vi "Calibration.vi"() -> ()   [LabVIEW 2021]
uses:
  C:/Users/User/Documents/CB III control files/Thorlabs.MotionControl.Controls.dll
  CB III control files/Thorlabs.MotionControl.Controls.dll
  C:/Users/User/Documents/CB III control files/ThorLabs.MotionControl.Benchtop.DCServoCLI.dll
  CB III control files/ThorLabs.MotionControl.Benchtop.DCServoCLI.dll
  C:/Users/User/Documents/CB III control files/ThorLabs.MotionControl.KCube.DCServoCLI.dll
  CB III control files/ThorLabs.MotionControl.KCube.DCServoCLI.dll
  C:/Users/User/Documents/CB III control files/Thorlabs.MotionControl.IntegratedStepperMotorsCLI.dll
  CB III control files/Thorlabs.MotionControl.IntegratedStepperMotorsCLI.dll
  <vilib>/Utility/file.llb/Read Delimited Spreadsheet (DBL).vi
  <vilib>/Utility/file.llb/Write Delimited Spreadsheet (DBL).vi
  <vilib>/ptbypt/NI_PtbyPt.lvlib
panel:
  in  "Drill camera#":dbl=1.0
  in  "OCT camera#":dbl=2.0
  out "sensitivity":dbl
  out "pilot_radii":dbl[][](array[numeric])
  out "pilot_centers":dbl[][](array[numeric])
  out "Targets in OCT":dbl[][](array[numeric])
  in  "take pic":bool
  out "Lumedica report 3":string
  in  "saveing method 3":string(combo)="SaveQueueImages"
  in  "USB camera calibration":bool
  out "OCT ON":bool=TRUE
  out "Lumedica report":string
  in  "saveing method":string(combo)="SaveQueueImages"
  in  "?":bool
  out "OCT imaging position":dbl[](array[numeric])
  in  "?":bool
  out "all pilot points":dbl[][](array[numeric])
  in  "Relative pilot points path":path=path "C:/Users/User/Documents/CB III control files/pilotpoints2.txt"
  in  "?":bool
  out "X-stage Control":refnum<k24>
  out "X stage properties":refnum<k24>
  in  "LongTravelStageControl":refnum<k24>(container)
  out "Zero Position":dbl[](array[numeric])
  out "Drill-Z-stage Control":refnum<k24>
  out "OCT-Z-stage-control":refnum<k24>
  out "Y-stage Control":refnum<k24>
  out "Y-stage properties":refnum<k24>
  out "Driller-Z-stage-Properties":refnum<k24>
  out "OCT-Z stage-properites":refnum<k24>
  in  "Trajectory":dbl[][](array[numeric])
  out "Velocity":T1(graph)
  out "position":T1(graph)
  in  "Driller Z- stage":refnum<k24>(container)
  in  "Y stage":refnum<k24>(container)
  in  "OCT Z-stage":refnum<k24>(container)
  # "USB Camera calibration"
  # "Constant trench depth on skull updates"
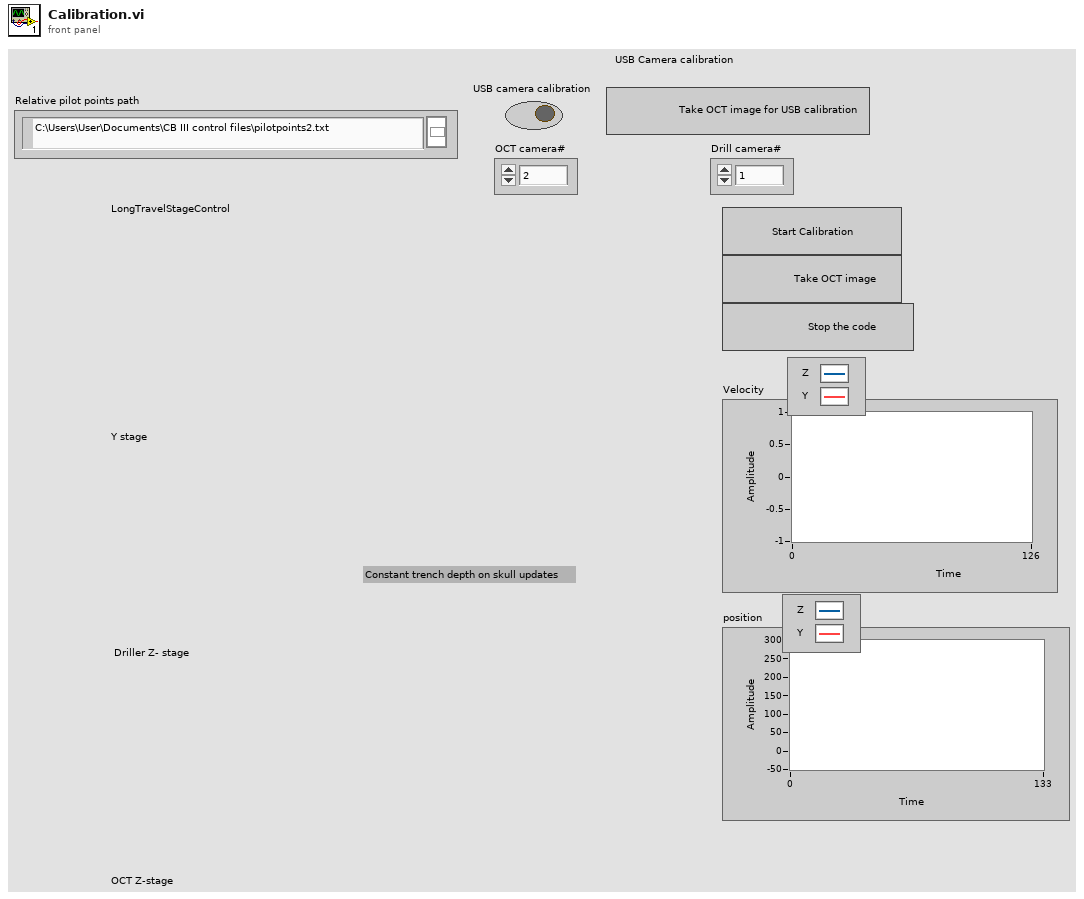
[diagram p1: front panel]
types:
  T1 = cluster{"[0]":dbl, "[1]":dbl, "[2]":dbl, "[3]":dbl, "[4]":dbl, "[5]":dbl, "[6]":dbl, "[7]":dbl, "[8]":dbl}
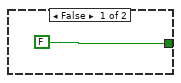
[diagram p3: hidden frame]
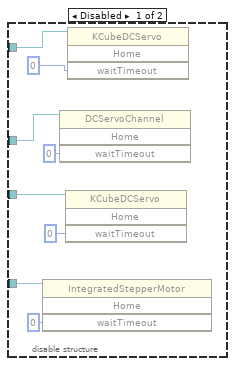
[diagram p4: hidden frame]
diagram:
  n1 = flat-sequence {
    tunnel: [w78] -> w5
    tunnel: w5 -> [w93]
    tunnel: [w211] -> w2
    tunnel: w2 -> [w216]
    tunnel: [w223] -> w4
    tunnel: [w222] -> w3
    tunnel: w4 -> [w225]
    tunnel: w3 -> [w224]
    frame #0 {
      # "Initiate all actuators"
      # "Initiate all actuators"
      n2 = property class="KCubeDCServoControl"(reference="Driller Z- stage", "SerialNumber"="27260819") -> (reference out=w39:refnum<k24>)  [unwired: 1 in, 1 out]
      n3 = property class="LongTravelStageControl"(reference="LongTravelStageControl", "SerialNumber"="45285094") -> (reference out=w28:refnum<k24>)  [unwired: 1 in, 1 out]
      n4 = property class="BenchtopDCServoControl"(reference="Y stage", "SerialNumber"="105278474") -> (reference out=w36:refnum<k24>)  [unwired: 1 in, 1 out]
      n5 = property class="KCubeDCServoControl"(reference="OCT Z-stage", "SerialNumber"="27261776") -> (reference out=w43:refnum<k24>)  [unwired: 1 in, 1 out]
      n6 = invoke class="KCubeDCServoControl" method="CreateDevice"(reference=w39) -> (reference out=w20:refnum<k24>)  [unwired: 2 in, 2 out]
      n7 = invoke class="LongTravelStageControl" method="CreateDevice"(reference=w28) -> (reference out=w27:refnum<k24>)  [unwired: 2 in, 2 out]
      n8 = invoke class="KCubeDCServoControl" method="CreateDevice"(reference=w43) -> (reference out=w18:refnum<k24>)  [unwired: 2 in, 2 out]
      n9 = invoke class="BenchtopDCServoControl" method="CreateDevice"(reference=w36) -> (reference out=w34:refnum<k24>)  [unwired: 2 in, 2 out]
      n10 = property class="KCubeDCServoControl"(reference=w18) -> (reference out=w33:refnum<k24>, "Device"=w16:refnum<k24>)  [unwired: 1 in, 1 out]
      n11 = local write "OCT-Z stage-properites"(w33) -> ()
      n12 = property class="LongTravelStageControl"(reference=w27) -> (reference out=w26:refnum<k24>, "Device"=w25:refnum<k24>)  [unwired: 1 in, 1 out]
      n13 = invoke class="IntegratedStepperMotor" method="SetBacklash"(reference=w25, "backlash"=0.002) -> ()  [unwired: 2 in, 4 out]
      n14 = property class="KCubeDCServoControl"(reference=w20) -> (reference out=w32:refnum<k24>, "Device"=w17:refnum<k24>)  [unwired: 1 in, 1 out]
      n15 = property class="BenchtopDCServoControl"(reference=w34) -> (reference out=w31:refnum<k24>, "BenchtopDCServo"=w23:refnum<k24>)  [unwired: 1 in, 1 out]
      n16 = invoke class="DCServoChannel" method="SetBacklash"(reference=w23, "backlash"=0.0) -> ()  [unwired: 2 in, 4 out]
      n17 = invoke class="IntegratedStepperMotor" method="EnableDevice"(reference=w25) -> ()  [unwired: 2 in, 3 out]
      n18 = invoke class="DCServoChannel" method="EnableDevice"(reference=w23) -> ()  [unwired: 2 in, 3 out]
      n19 = invoke class="KCubeDCServo" method="SetBacklash"(reference=w17, "backlash"=0.007) -> ()  [unwired: 2 in, 4 out]
      n20 = invoke class="KCubeDCServo" method="SetBacklash"(reference=w16, "backlash"=0.007) -> ()  [unwired: 2 in, 4 out]
      n21 = local write "OCT-Z-stage-control"(w16) -> ()
      n22 = local write "Driller-Z-stage-Properties"(w32) -> ()
      n23 = local write "Drill-Z-stage Control"(w17) -> ()
      n24 = local write "X stage properties"(w26) -> ()
      n25 = local write "X-stage Control"(w25) -> ()
      n26 = local write "Y-stage properties"(w31) -> ()
      n27 = local write "Y-stage Control"(w23) -> ()
    }
    frame #1 {
      # "Home actuators"
      n28 = local read "Drill-Z-stage Control"() -> (w47:refnum<k24>)
      n29 = local read "OCT-Z-stage-control"() -> (w45:refnum<k24>)
      n30 = local read "Y-stage Control"() -> (w46:refnum<k24>)
      n31 = local read "X-stage Control"() -> (w44:refnum<k24>)
      n32 = disable-structure shown="Enabled" {
        disable-tunnel: w46 -> [w55 _]
        disable-tunnel: w47 -> [w53 _]
        disable-tunnel: w45 -> [w51 _]
        disable-tunnel: w44 -> [w49 _]
        frame Disabled {
          n33 = invoke class="IntegratedStepperMotor" method="Home"(reference=w49, "waitTimeout"=0) -> ()  [unwired: 2 in, 4 out]
          n34 = invoke class="DCServoChannel" method="Home"(reference=w55, "waitTimeout"=0) -> ()  [unwired: 2 in, 4 out]
          n35 = invoke class="KCubeDCServo" method="Home"(reference=w51, "waitTimeout"=0) -> ()  [unwired: 2 in, 4 out]
          n36 = invoke class="KCubeDCServo" method="Home"(reference=w53, "waitTimeout"=0) -> ()  [unwired: 2 in, 4 out]
        }
        frame Enabled {
        }
      }
    }
    frame #2 {
      n37 = case shown="True" "USB camera calibration" {
        frame False {
        }
        frame True {
          n38 = flat-sequence {
            frame #0 {
              n39 = local write "OCT ON"(TRUE ("OCT ON")) -> ()
              n40 = Wait (ms)(milliseconds to wait=u32 3000) -> ()  [unwired: 1 out]
            }
            frame #1 {
              n41 = script code="crop_pixels=100;\nvid = videoinput('winvideo',OCT_cam);\nvidInfo = imaqhwinfo(vid);\nvidRes = vid.VideoResolution;\nnBands = vid.NumberOfBands; \nhFig=figure('Renderer', 'painters', 'Position', [1200 200 vidRes(1)/2 vidRes(2)-crop_pixels]);\nhAxes = axes(hFig);\nhImage = image(hAxes, zeros(vidRes(2)-crop_pixels, vidRes(1)/2, nBands)); \nsetappdata(hImage,'UpdatePreviewWindowFcn',@mypreview_fnc);\npreview(vid, hImage); \n% adding the OCT image boarders to the video\nhold on\ntext(-40,-35,'Make sure you have chosen correct camera as OCT camera. if not, stop and change the #','FontWeight','bold','FontSize',12)\nclear camObject;"("OCT_cam"="OCT camera#") -> ()  [unwired: 1 in, 1 out]
            }
            frame #2 {
              n42 = while {
                stop <- "take pic" stop-if-true
              }
              n43 = local write "OCT ON"(FALSE ("OCT ON")) -> ()
            }
            frame #3 {
              n44 = call "OCT_Run_sub.vi"("saveing method"="saveing method 3") -> ("Lumedica report"=→"Lumedica report 3":string)  [unwired: 10 in]
            }
            frame #4 {
              n45 = script code="close all"() -> ()  [unwired: 1 in, 1 out]
              n46 = call <vilib>:"System Exec.vi"("run minimized? (F)"=TRUE, "wait until completion? (T)"=TRUE, "command line"="cmd /c taskkill /IM OctEngine.exe") -> ()  [unwired: 5 in, 4 out]
            }
            frame #5 {
              n47 = call <vilib>:"Application Directory.vi"() -> ("Application Directory"=w69:path)
              n48 = local read "OCT camera#"() -> (w67:dbl)
              n49 = script code="% %% Finding and reading the OCT scans\ndirc = dir(Path);\ndirc = dirc(find(~cellfun(@isdir,{dirc(:).name})));\n[A,I] = max([dirc(:).datenum]);\nif ~isempty(I)\n    latestfile = dirc(I).name;\nend\n\n% finding the surface \ndims=[512 512 512]; \n% path to the images just taken\nfPath=[Path,'\\',latestfile,'\\'];\n%the files name starts with:\nfScanName='BSCAN-SGL';\n%%%%%%%%%%%%%%%%  Surface detecton + cleaning %%%%%%%%%%%%%%%%\n\n% Import scans\nvol=zeros(dims);\nfor k=1:dims(3)\n    %%% Import volume\n    fNameTemp=join([fPath,fScanName,'-',num2str(sprintf('%03d',k)),'.tif']);\n    imTemp=imread(fNameTemp);\n    vol(:,:,k)=imTemp(:,:,1); % convert to grayscale, taking only first channel\nend\n\n%%%% Construct top view image %%%%\nimRecon=reshape(sum(vol,1),512,512);\nclear vol\nimRecon=imadjust(rescale(imRecon)); % Initial rescale from [0,1] and contrast increase\n\n% calculate ranges for contrast shifting based on mean +/- stdev\nimAve=mean2(imRecon); imStdev=std2(imRecon); \nn=3; % set ranges to n stdevs above & below mean\nif imAve-n*imStdev<0 % min must not be below zero\n    rngMin=0;\nelse\n    rngMin=imAve-n*imStdev;\nend\nif imAve+n*imStdev>1 % max must not be above 1\n    rngMax=1;\nelse\n    rngMax=imAve+n*imStdev;\nend\nclear imStdev imAve\n\n% smooth contrast, preserving strong edges\nedgeThresh=0.1; amnt=-0.8; \nimRecon=localcontrast(single(imRecon),edgeThresh,amnt); \n\n% adjust contrast range again & curve to lighten images\ngamma=0.6; \nimTopView=imadjust(imRecon,[rngMin rngMax],[],gamma); \nclear imRecon\n\n% correct orientation for consistency with other plots  \nimTopView=imTopView(end:-1:1,end:-1:1)';\n\n%%WEbcam calibration\n%path='C:\\Users\\Lumedica\\Documents\\CB III Kinesis\\';\nclc\ncam = webcam(2);\nimg = snapshot(cam); % snapshot of the webcam\nimg=rot90(img(:,end/2:end,:),-1);\nimage=figure;\nsubplot(1,2,2)\nimshow(imTopView)\nsubplot(1,2,1)\nimshow(img);\npoints=drawpolygon;\npilot=points.Position;\nclose(image)\nclosePreview(cam)\nsave([path,'\\pilot.mat'],'pilot','OCT_cam','Drill_cam')\nclear camObject;"("Path"=path "C:/Users/Public/Documents/Lumedica/OctEngine/Data" ("file path (dialog if empty)"), "path"=w69, "OCT_cam"=w67, "Drill_cam"="Drill camera#") -> ()  [unwired: 1 in, 1 out]
            }
            frame #6 {
              n50 = Stop(stop? (T)=TRUE) -> ()
            }
          }
        }
      }
    }
    frame #3 {
      # "pick a holistic Z value to start calibration\nThis does not need to be accurate but needs \nto be close enough"
      n51 = while {
        tunnel: [w84] -> w75
        tunnel: [w82] -> w74
        tunnel: [w80] -> w78
        stop <- "?" stop-if-true
        n52 = local read "Drill-Z-stage Control"() -> (w81:refnum<k24>)
        n53 = local read "Y-stage Control"() -> (w83:refnum<k24>)
        n54 = local read "X-stage Control"() -> (w85:refnum<k24>)
        n55 = Wait (ms)(milliseconds to wait=u32 20) -> ()  [unwired: 1 out]
        n56 = call "Y_absolute_position.vi"(".NET Refnum in"=w83) -> ("Numeric"=w82:dbl)  [unwired: 9 in, 1 out]
        n57 = call "Z_absolute_position.vi"(".NET Refnum in"=w81) -> ("Numeric"=w80:dbl)  [unwired: 9 in, 1 out]
        n58 = call "X-absolute_position.vi"(".NET Refnum in"=w85) -> ("Numeric"=w84:dbl)  [unwired: 9 in, 1 out]
      }
      n59 = One Button Dialog(message="Move the driller tip to the same sample point you like ( in the center of the sample). lower the drillbit into sample just a bit. \nclick \"Start Calibration\"when you are done ", button name ("OK")="OK") -> ()  [unwired: 1 out]
      n60 = Build Array(w75, w74, w78, 0.0 ("element")) -> (w73:dbl[])
      n61 = local write "Zero Position"(w73) -> ()
    }
    frame #4 {
      w89 = 1.0 ("maxVelocity")
      # "Getting ready to start drilling the pilot points"
      n62 = local read "Drill-Z-stage Control"() -> (w90:refnum<k24>)
      n63 = while {
        stop <- w96 stop-if-true
        n64 = One Button Dialog(message="Ready for generating pilot points?", button name ("OK")="Yes!") -> (true=w96:bool)
      }
      n65 = Subtract(x=w93, y=2.0) -> (x-y=w87:dbl)
      n66 = call-poly <vilib>:"Read Delimited Spreadsheet.vi"("file path (dialog if empty)"="Relative pilot points path") -> ("all rows"=w91:dbl[][])  [unwired: 9 in, 5 out]
      n67 = local write "all pilot points"(w91) -> ()
      n68 = call "motion control_Z.vi"("position"=w87, "acceleration"=w89, "maxVelocity"=w89, ".NET Refnum in"=w90) -> ()  [unwired: 1 in, 1 out]
    }
    frame #5 {
      # "Drilling holes one by one and move to the next"
      n69 = local read "all pilot points"() -> (w103:dbl[][])
      n70 = Array Size(array=w103) -> (size(s)=w106:i32[])
      n71 = Transpose 2D Array(2D array=w103) -> (transposed array=w102:dbl[][])
      n72 = Index Array(array=w106, index=1) -> (element=w105:i32)
      n73 = for {
        N: w105 -> [_]
        tunnel: w102 -> [w111] mode=indexing
        tunnel: [w110] -> w101 mode=indexing
        n74 = local read "Zero Position"() -> (w118:dbl[])
        n75 = flat-sequence {
          tunnel: w109 -> [w125]
          tunnel: w108 -> [w124]
          tunnel: w107 -> [w127]
          tunnel: w107 -> [w132]
          frame #0 {
            w122 = 3.0 ("acceleration")
            w123 = 3.0 ("acceleration")
            n76 = local read "Y-stage Control"() -> (w120:refnum<k24>)
            n77 = local read "X-stage Control"() -> (w121:refnum<k24>)
            n78 = call "Motion_control_X.vi"(".NET Refnum in"=w121, "maxVelocity"=w122, "acceleration"=w122, "position"=w125) -> ()  [unwired: 6 in, 1 out]
            n79 = call "motion_control.vi"("position"=w124, "acceleration"=w123, "maxVelocity"=w123, ".NET Refnum in"=w120) -> ()  [unwired: 1 in, 1 out]
            n80 = Wait (ms)(milliseconds to wait=u32 100) -> ()  [unwired: 1 out]
          }
          frame #1 {
            w128 = 3.0 ("maxVelocity")
            n81 = local read "Drill-Z-stage Control"() -> (w129:refnum<k24>)
            n82 = call "motion control_Z.vi"("position"=w127, "acceleration"=w128, "maxVelocity"=w128, ".NET Refnum in"=w129) -> ()  [unwired: 1 in, 1 out]
            n83 = Wait (ms)(milliseconds to wait=u32 100) -> ()  [unwired: 1 out]
          }
          frame #2 {
            w134 = 3.0 ("maxVelocity")
            n84 = local read "Drill-Z-stage Control"() -> (w135:refnum<k24>)
            n85 = Subtract(x=w132, y=3.0) -> (x-y=w133:dbl)
            n86 = call "motion control_Z.vi"("position"=w133, "acceleration"=w134, "maxVelocity"=w134, ".NET Refnum in"=w135) -> ()  [unwired: 1 in, 1 out]
            n87 = Wait (ms)(milliseconds to wait=u32 100) -> ()  [unwired: 1 out]
          }
        }
        n88 = Add(x=w111, y=w118) -> (x+y=w117:dbl[])
        n89 = Index Array(array=w117, index #1=0 ("index"), index #2=1 ("index"), index #3=2 ("index"), index #4=3 ("index")) -> (element #1=w109:dbl, element #2=w108:dbl, element #3=w107:dbl, element #4=w112:dbl)
        n90 = Build Array(w109, w108, w107, w112) -> (w110:dbl[])
      }
      n91 = call <vilib>:"Application Directory.vi"() -> ("Application Directory"=w98:path)
      n92 = Build Path(base path=w98, name or relative path=path "Generated_calibration_points.txt") -> (appended path=w99:path)
      n93 = Transpose 2D Array(2D array=w101) -> (transposed array=w100:dbl[][])
      n94 = call-poly <vilib>:"Write Delimited Spreadsheet.vi"("file path (dialog if empty)"=w99, "2D data"=w100) -> ()  [unwired: 12 in, 2 out]
    }
    frame #6 {
      w137 = 3.0 ("maxVelocity")
      # "Dont zero the driller due to\n zeroing issue with the actuator"
      # "Get the driller out of the way"
      n95 = local read "Drill-Z-stage Control"() -> (w138:refnum<k24>)
      n96 = call "motion control_Z.vi"("position"=1.0, "acceleration"=w137, "maxVelocity"=w137, ".NET Refnum in"=w138) -> ()  [unwired: 1 in, 1 out]
    }
    frame #7 {
      w141 = 20.0 ("maxVelocity")
      # "Go to OCT stage"
      n97 = local read "X-stage Control"() -> (w145:refnum<k24>)
      n98 = local read "Y-stage Control"() -> (w144:refnum<k24>)
      n99 = call "Motion_control_X.vi"(".NET Refnum in"=w145, "maxVelocity"=w141, "acceleration"=w141, "position"=280.0) -> ()  [unwired: 6 in, 1 out]
      n100 = call "motion_control.vi"("position"=4.4, "acceleration"=5.0, "maxVelocity"=2.5, ".NET Refnum in"=w144) -> ()  [unwired: 1 in, 1 out]
    }
    frame #8 {
      # "Open the USB video camera to adjust the sample under OCT"
      n101 = call <vilib>:"Application Directory.vi"() -> ("Application Directory"=w146:path)
      n102 = script code="load([path,'\\pilot.mat'])\ncrop_pixels=100;\nvid = videoinput('winvideo',OCT_cam);\nvidInfo = imaqhwinfo(vid);\nvidResu = vid.VideoResolution;\nnBandss = vid.NumberOfBands; \nhFig=figure('Renderer', 'painters', 'Position', [1200 200 vidResu(1)/2 vidResu(2)-crop_pixels]);\nhAxes1 = axes(hFig)\nhImage = image(axes(hFig), zeros(vidResu(2)-crop_pixels, vidResu(1)/2, nBandss)); \nsetappdata(hImage,'UpdatePreviewWindowFcn',@mypreview_fnc);\npreview(vid, hImage); \n% adding the OCT image boarders to the video\nhold on\ntext(-40,-35,'Make sure your ROI is in the green rectangle. if it is, just close the window','FontWeight','bold','FontSize',12)\nline([pilot(1,1) pilot(2,1)], [pilot(1,2) pilot(2,2)],'Color','g','LineWidth',3);\nline([pilot(2,1) pilot(3,1)], [pilot(2,2) pilot(3,2)],'Color','g','LineWidth',3);\nline([pilot(3,1) pilot(4,1)], [pilot(3,2) pilot(4,2)],'Color','g','LineWidth',3);\nline([pilot(4,1) pilot(1,1)], [pilot(4,2) pilot(1,2)],'Color','g','LineWidth',3);\n\nclear camObject;"("path"=w146) -> ()  [unwired: 1 in, 1 out]
    }
    frame #9 {
      # "Open lumedica"
      n103 = while {
        stop <- w151 stop-if-true
        n104 = One Button Dialog(message="Adjust the sample position under the scanner and hit \"Take OCT image\" in labview", button name ("OK")="OK") -> (true=w151:bool)
      }
      n105 = while {
        stop <- "?" stop-if-true
      }
      n106 = local write "OCT ON"(TRUE ("OCT ON")) -> ()
    }
    frame #10 {
      # "take the OCT image"
      n107 = script code="close all"() -> ()  [unwired: 1 in, 1 out]
      n108 = local write "OCT ON"(FALSE ("OCT ON")) -> ()
      n109 = call "OCT_Run_sub.vi"("saveing method"="saveing method") -> ("Lumedica report"=→"Lumedica report":string)  [unwired: 10 in]
    }
    frame #11 {
      # "Close lumedica"
      n110 = call <vilib>:"System Exec.vi"("run minimized? (F)"=TRUE, "wait until completion? (T)"=TRUE, "command line"="cmd /c taskkill /IM OctEngine.exe") -> ()  [unwired: 5 in, 4 out]
    }
    frame #12 {
      # "Calculate the affine transfer matrix and specify target points for sanity check"
      n111 = call <vilib>:"Application Directory.vi"() -> ("Application Directory"=w159:path)
      n112 = while {
        tunnel: [w176] -> w167
        tunnel: [w175] -> w166
        tunnel: [w174] -> w165
        tunnel: [w173] -> w164
        tunnel: [w172] -> w163
        i -> [w177]
        stop <- w171 stop-if-true
        n113 = Multiply(x=0.05 ("y"), y=w177) -> (x*y=w179:dbl)
        n114 = Subtract(x=0.9, y=w179) -> (x-y=w170:dbl)
        n115 = local write "sensitivity"(w170) -> ()
        n116 = flat-sequence {
          tunnel: w170 -> [w186]
          tunnel: [w185] -> w176
          tunnel: [w184] -> w175
          tunnel: [w183] -> w174
          tunnel: [w182] -> w173
          tunnel: [w181] -> w172
          tunnel: [w187] -> w171
          frame #0 {
            n117 = script code="%% finding the pilot holes\n% Correct the last recorded image\nPath='C:\\Users\\Public\\Documents\\Lumedica\\OctEngine\\Data';\nlatestfile = find_latestfile(Path);\nvol=Full_correct_C([Path,'\\',latestfile]);\n% S_H_detect is a functio that I use to find the surface and the drilled holes on it\n[centers,radii,depth,dorsal_surface,im]=S_H_detect_C(sensetivity,vol);\nclose all"("sensetivity"=w186) -> ("centers"=w182:dbl[][], "radii"=w181:dbl[][], "depth"=w183:dbl[], "dorsal_surface"=w184:dbl[][], "im"=w185:dbl[][])  [unwired: 1 in, 1 out]
          }
          frame #1 {
            n118 = Two Button Dialog(message="Are you happy with the detected circles?", 1:"Nope!" ("F button name (\"Cancel\")"), 2:"Yes" ("T button name (\"OK\")")) -> (T button?=w187:bool)
          }
        }
      }
      n119 = script code="Rdir=[rdir,'\\'];\n% Generate the transformation matrix\n%Genrate pilot point positios in the OCT as n rows of [X, Y Z ,1]\ncenters_all=[centers depth' ones(length(depth),1)];\npoints=importdata([Rdir,'Generated_calibration_points.txt'])';   % points read by the drillers axis\n% load('Best_points.mat','BC');\n% points=BC;\n% X=points(1,1)-points2(1,1);\n% Y=points(1,2)-points2(1,2);\n% Z=points(1,3)-points2(1,3);\n% points2=[points2(:,1)+X,points2(:,2)+Y,points2(:,3)+Z,points2(:,4)];\n% points=points2;\n% points2=BC;\n% Normalize the problem:    \n%For world:\nAu=mean(points(:,1));\nAv=mean(points(:,2));\nAw=mean(points(:,3));\ns=length(points)*sqrt(3)/sum(((Au-points(:,1)).^2+(Av-points(:,2)).^2+(Aw-points(:,3)).^2).^0.5);\nT=s*[1 0 0 -Au;0 1 0 -Av;0 0 1 -Aw;0 0 0 1/s];\n% Normalize the pilot points:\nN_points=points*T;\n\n\n% For OCT:\nAup=mean(centers_all(:,1));\nAvp=mean(centers_all(:,2));\nAwp=mean(centers_all(:,3));\ns=length(centers_all)*sqrt(3)/sum(((Aup-centers_all(:,1)).^2+(Avp-centers_all(:,2)).^2+(Awp-centers_all(:,3)).^2).^0.5);\nTp=s*[1 0 0 -Aup;0 1 0 -Avp;0 0 1 -Awp;0 0 0 1/s];\nN_centers_all=centers_all*Tp;\n\n% Find the transfer matrix\n H_hat=N_centers_all\\N_points;\n OCT2World=Tp*H_hat/T;\n%OCT2World=centers_all\\points2; % left side multiply the transformation matrix\nwritematrix(OCT2World,[Rdir,'calibration_matrix.txt'],'Delimiter','tab') % save the calibration matrix\n\n% selsct test points to check the calibration\nfigure\n imshow(im);\n title('select the target points for sanity check, press enter in the end')\n % Draw the previouse holes\nviscircles(centers,radii,'LineWidth',0.4);\n[X,Y]=getpts; % select target points for drilling\n% X=[202;342;360;234];\n% Y=[192;195;307;335];\nC=[round(X),round(Y)];  \n% test=readmatrix('C:\\Users\\User\\Documents\\CB III control files\\calibration_matrix.txt');\n% Draw the nre targets and give them depth\nlen=length(X);\nW=zeros(len,4);\npt=W;\nfor i=1:len\n    viscircles([X(i),Y(i)],radii(1),'LineWidth',0.4,'Color','b')\n    %the depth of each point would be random value between 10 to 25 pixcels down from the surface\n    pt(i,:)=[round(X(i));round(Y(i));dorsal_surface(round(Y(i)),round(X(i)))-round(10+30*rand(1));1]'; \n    % Calculate the coordinate of trget points in the driller space\n    W(i,:)=pt(i,:)*OCT2World;\n  %  W2(i,:)=pt(i,:)*test;\nend\n\n% save the test point coordinates for drilling\nwritematrix(W,[Rdir,'test_points.txt'],'Delimiter','tab')"("centers"=w164, "radii"=w163, "depth"=w165, "dorsal_surface"=w166, "im"=w167, "rdir"=w159) -> ("pt"=w168:dbl[][], "centers"=w162:dbl[][], "radii"=w169:dbl[][])  [unwired: 1 in, 1 out]
      n120 = call <vilib>:"Application Directory.vi"() -> ("Application Directory"=w158:path)
      n121 = Build Path(base path=w158, name or relative path=path "Cal_read_centers.txt") -> (appended path=w160:path)
      n122 = local write "Targets in OCT"(w168) -> ()
      n123 = local write "pilot_radii"(w169) -> ()
      n124 = call-poly <vilib>:"Write Delimited Spreadsheet.vi"("file path (dialog if empty)"=w160, "2D data"=w162) -> ()  [unwired: 12 in, 2 out]
      n125 = local write "pilot_centers"(w162) -> ()
    }
    frame #13 {
      # "Record the robot position during imaging"
      n126 = call <vilib>:"Application Directory.vi"() -> ("Application Directory"=w193:path)
      n127 = local read "OCT-Z-stage-control"() -> (w194:refnum<k24>)
      n128 = local read "X-stage Control"() -> (w195:refnum<k24>)
      n129 = local read "Y-stage Control"() -> (w196:refnum<k24>)
      n130 = call "X-absolute_position.vi"(".NET Refnum in"=w195) -> ("Numeric"=w197:dbl)  [unwired: 9 in, 1 out]
      n131 = call "Y_absolute_position.vi"(".NET Refnum in"=w196) -> ("Numeric"=w198:dbl)  [unwired: 9 in, 1 out]
      n132 = call "Z_absolute_position.vi"(".NET Refnum in"=w194) -> ("Numeric"=w199:dbl)  [unwired: 9 in, 1 out]
      n133 = Build Path(base path=w193, name or relative path=path "Calibration_imaging_position.txt") -> (appended path=w191:path)
      n134 = Build Array(w197, w198, w199) -> (w200:dbl[])
      n135 = local write "OCT imaging position"(w200) -> ()
      n136 = call-poly <vilib>:"Write Delimited Spreadsheet.vi"("file path (dialog if empty)"=w191, "1D data"=w200) -> ()  [unwired: 12 in, 2 out]
    }
    frame #14 {
      w207 = 20.0 ("maxVelocity")
      w208 = 3.0 ("maxVelocity")
      # "Move back the stage to driller"
      n137 = local read "X-stage Control"() -> (w210:refnum<k24>)
      n138 = local read "Y-stage Control"() -> (w209:refnum<k24>)
      n139 = local read "Zero Position"() -> (w206:dbl[])
      n140 = Index Array(array=w206, index #1=0 ("index"), index #2=1 ("index"), index #3=2 ("index")) -> (element #1=w203:dbl, element #2=w202:dbl, element #3=w211:dbl)
      n141 = call "Motion_control_X.vi"(".NET Refnum in"=w210, "maxVelocity"=w207, "acceleration"=w207, "position"=w203) -> ()  [unwired: 6 in, 1 out]
      n142 = call "motion_control.vi"("position"=w202, "acceleration"=w208, "maxVelocity"=w208, ".NET Refnum in"=w209) -> ()  [unwired: 1 in, 1 out]
    }
    frame #15 {
      w215 = 3.0 ("acceleration")
      # "fast bring down the driller"
      n143 = local read "Drill-Z-stage Control"() -> (w214:refnum<k24>)
      n144 = Subtract(x=w216, y=5.0) -> (x-y=w213:dbl)
      n145 = call "motion control_Z.vi"("position"=w213, "acceleration"=w215, "maxVelocity"=w215, ".NET Refnum in"=w214) -> ()  [unwired: 1 in, 1 out]
    }
    frame #16 {
      # "Read the expected points"
      n146 = call <vilib>:"Application Directory.vi"() -> ("Application Directory"=w219:path)
      n147 = Build Path(base path=w219, name or relative path=path "test_points.txt") -> (appended path=w217:path)
      n148 = call-poly <vilib>:"Read Delimited Spreadsheet.vi"("file path (dialog if empty)"=w217) -> ("all rows"=w222:dbl[][])  [unwired: 9 in, 5 out]
      n149 = Array Size(array=w222) -> (size(s)=w221:i32[])
      n150 = Index Array(array=w221, index=0) -> (element=w223:i32)
    }
    frame #17 {
      # "Drill the expected points in the sample"
      n151 = for {
        N: w225 -> [_]
        tunnel: w224 -> [w233] mode=indexing
        n152 = flat-sequence {
          tunnel: w229 -> [w235]
          tunnel: w228 -> [w234]
          tunnel: w227 -> [w241]
          tunnel: [w241] -> w226
          tunnel: w226 -> [w246]
          frame #0 {
            w236 = 3.0 ("maxVelocity")
            w237 = 3.0 ("maxVelocity")
            n153 = local read "X-stage Control"() -> (w238:refnum<k24>)
            n154 = local read "Y-stage Control"() -> (w239:refnum<k24>)
            n155 = call "motion_control.vi"("position"=w234, "acceleration"=w236, "maxVelocity"=w236, ".NET Refnum in"=w239) -> ()  [unwired: 1 in, 1 out]
            n156 = call "Motion_control_X.vi"(".NET Refnum in"=w238, "maxVelocity"=w237, "acceleration"=w237, "position"=w235) -> ()  [unwired: 6 in, 1 out]
            n157 = Wait (ms)(milliseconds to wait=u32 100) -> ()  [unwired: 1 out]
          }
          frame #1 {
            w243 = 3.0 ("maxVelocity")
            n158 = local read "Drill-Z-stage Control"() -> (w244:refnum<k24>)
            n159 = call "motion control_Z.vi"("position"=w241, "acceleration"=w243, "maxVelocity"=w243, ".NET Refnum in"=w244) -> ()  [unwired: 1 in, 1 out]
            n160 = Wait (ms)(milliseconds to wait=u32 100) -> ()  [unwired: 1 out]
          }
          frame #2 {
            w249 = 3.0 ("maxVelocity")
            n161 = local read "Drill-Z-stage Control"() -> (w250:refnum<k24>)
            n162 = Subtract(x=w246, y=1.2) -> (x-y=w245:dbl)
            n163 = call "motion control_Z.vi"("position"=w245, "acceleration"=w249, "maxVelocity"=w249, ".NET Refnum in"=w250) -> ()  [unwired: 1 in, 1 out]
            n164 = Wait (ms)(milliseconds to wait=u32 100) -> ()  [unwired: 1 out]
          }
        }
        n165 = Index Array(array=w233, index #1=0 ("index"), index #2=1 ("index"), index #3=2 ("index")) -> (element #1=w229:dbl, element #2=w228:dbl, element #3=w227:dbl)
      }
    }
    frame #18 {
      w251 = 2.0 ("maxVelocity")
      n166 = while {
        stop <- w256 stop-if-true
        n167 = One Button Dialog(message="Going back for sanity check", button name ("OK")="OK") -> (true=w256:bool)
      }
      n168 = local read "Drill-Z-stage Control"() -> (w253:refnum<k24>)
      n169 = call "motion control_Z.vi"("position"=1.0, "acceleration"=w251, "maxVelocity"=w251, ".NET Refnum in"=w253) -> ()  [unwired: 1 in, 1 out]
    }
    frame #19 {
      w258 = 1.0 ("maxVelocity")
      w261 = 1.0 ("acceleration")
      w264 = 20.0 ("maxVelocity")
      # "Go back to OCT station"
      n170 = local read "Y-stage Control"() -> (w260:refnum<k24>)
      n171 = local read "OCT imaging position"() -> (w266:dbl[])
      n172 = local read "OCT-Z-stage-control"() -> (w259:refnum<k24>)
      n173 = Index Array(array=w266, index #1=0 ("index"), index #2=1 ("index"), index #3=2 ("index")) -> (element #1=w263:dbl, element #2=w262:dbl, element #3=w257:dbl)
      n174 = local read "X-stage Control"() -> (w265:refnum<k24>)
      n175 = call "motion control_Z.vi"("position"=w257, "acceleration"=w258, "maxVelocity"=w258, ".NET Refnum in"=w259) -> ()  [unwired: 1 in, 1 out]
      n176 = call "Motion_control_X.vi"(".NET Refnum in"=w265, "maxVelocity"=w264, "acceleration"=w264, "position"=w263) -> ()  [unwired: 6 in, 1 out]
      n177 = call "motion_control.vi"("position"=w262, "acceleration"=w261, "maxVelocity"=w261, ".NET Refnum in"=w260) -> ()  [unwired: 1 in, 1 out]
    }
    frame #20 {
      # "open lumedica"
      n178 = local write "OCT ON"(TRUE ("OCT ON")) -> ()
      n179 = Wait (ms)(milliseconds to wait=u32 3000) -> ()  [unwired: 1 out]
    }
    frame #21 {
      # "take the new images"
      n180 = call "OCT_Run_sub.vi"() -> ()  [unwired: 11 in, 1 out]
      n181 = local write "OCT ON"(FALSE ("OCT ON")) -> ()
    }
    frame #22 {
      # "Close lumedica"
      n182 = call <vilib>:"System Exec.vi"("run minimized? (F)"=TRUE, "wait until completion? (T)"=TRUE, "command line"="cmd /c taskkill /IM OctEngine.exe") -> ()  [unwired: 5 in, 4 out]
    }
    frame #23 {
      # "Calculate the calibration Error"
      # ">>> I added clear all here, I hope it doesnt hurt!<<<<"
      n183 = local read "pilot_radii"() -> (w280:dbl[][])
      n184 = local read "Targets in OCT"() -> (w282:dbl[][])
      n185 = local read "sensitivity"() -> (w283:dbl)
      n186 = while {
        tunnel: [w290] -> w278
        tunnel: [w289] -> w277
        tunnel: [w288] -> w279
        tunnel: [w287] -> w276
        i -> [w291]
        stop <- w286 stop-if-true
        n187 = local read "sensitivity"() -> (w284:dbl)
        n188 = Multiply(x=0.05 ("y"), y=w291) -> (x*y=w293:dbl)
        n189 = Subtract(x=w284, y=w293) -> (x-y=w285:dbl)
        n190 = flat-sequence {
          tunnel: w285 -> [w298]
          tunnel: [w297] -> w290
          tunnel: [w296] -> w289
          tunnel: [w295] -> w288
          tunnel: [w294] -> w287
          tunnel: [w299] -> w286
          frame #0 {
            n191 = script code="%% finding the pilot holes\n% Correct the last recorded image\nPath='C:\\Users\\Public\\Documents\\Lumedica\\OctEngine\\Data';\nlatestfile = find_latestfile(Path);\nvol=Full_correct_C([Path,'\\',latestfile]);\n% S_H_detect is a functio that I use to find the surface and the drilled holes on it\n[centers,radii,depth,~,im]=S_H_detect_C(sensetivity,vol);\nclose all"("sensetivity"=w298) -> ("centers"=w295:dbl[][], "radii"=w294:dbl[][], "depth"=w296:dbl[], "im"=w297:dbl[][])  [unwired: 1 in, 1 out]
          }
          frame #1 {
            n192 = Two Button Dialog(message="Are you happy with the detected circles?", 1:"Nope!" ("F button name (\"Cancel\")"), 2:"Yes" ("T button name (\"OK\")")) -> (T button?=w299:bool)
          }
        }
      }
      n193 = local read "pilot_centers"() -> (w281:dbl[][])
      n194 = script code="imshow(im)\nhold on\n\nfor i=1:length(pt)\nviscircles(pt(i,1:2),radii(1),'LineWidth',0.4,'color','b') % the clicked circles\nend\nviscircles(centers,radii,'LineWidth',0.3,'color','k','LineStyle','--') % the old circles\n\n% remove the pilot points:\nclc\nindx=zeros(length(centers),1);\nfor m=1:length(centers) % length of the number of previous pilot points only\n    tt=sum(abs(centers_S-centers(m,:)),2); % find the distance of sll the new points from the pilot points\n    indx(m)=find(tt==min(tt)); % for each point find the new point with leat distanc e from the pilot point, record their indeise\nend\ncentersd=[centers_S depth_S']; % add depth to the found centers\ncentersd(indx,:)=[]; % remove the points that are just pilot points\nradiid=radii_S;\nradiid(indx,:)=[]; % remove the radii of the removed points\ncc2=[pt(:,1:2) pt(:,3)]; %expected points and expected depths \n\n%%% for the random placed points to be found correctly %%%\nerror=zeros(length(centersd),3);\nfor n=1:length(centersd)\n    tt=sum(abs(pt(:,1:2)-centersd(n,1:2)),2);\n    % find the closeset found hole to the target\n    ER=find(tt==min(tt));\n    error(n,:)=centersd(n,:)-cc2(ER,:);\nend\n% error=abs(cc2-centersd);\nLpixel=11;\nApixel=14;\nError=[error(:,1)*Lpixel error(:,2)*Lpixel error(:,3)*Apixel];\nfigure\nsubplot(2,1,1)\nboxplot(Error)\ntitle(['Error on differnt axis for ', num2str(length(cc2)),' points'])\nxlabel('Axis')\nylabel('Error (\\mum)')\nxticklabels({'X','Y','Z'})\n % Dot plot of the error magnetudes\n\nX=ones(length(Error),2);\nX(:,2)=Error(:,1);\nY=2*ones(length(Error),2);\nY(:,2)=Error(:,2);\nZ=3*ones(length(Error),2);\nZ(:,2)=Error(:,3);\nDindx=1:length(Error);\ntDindx=[Dindx';Dindx';Dindx'];\n\nall_pt=[X;Y;Z];\nsubplot(2,1,2)\ngscatter(all_pt(:,1),all_pt(:,2),tDindx,[],\"o\");\ntitle(['absolute Error on differnt axis for ', num2str(length(cc2)),' points'])\nxlabel('Axis')\nylabel('Error (\\mum)')\nb = gca; legend(b,'off');\nxticks([1 2 3])\nxticklabels({'X','Y','Z'})\nclear all"("radii"=w280, "centers"=w281, "pt"=w282, "sens"=w283, "centers_S"=w279, "radii_S"=w276, "depth_S"=w277, "im"=w278) -> ()  [unwired: 1 in, 1 out]
    }
    frame #24 {
      n195 = Stop(stop? (T)=TRUE) -> ()
    }
  }
  n196 = local read "OCT-Z stage-properites"() -> (w10:refnum<k24>)
  n197 = local read "OCT-Z stage-properites"() -> (w15:refnum<k24>)
  n198 = local read "X stage properties"() -> (w7:refnum<k24>)
  n199 = local read "Y-stage properties"() -> (w14:refnum<k24>)
  n200 = flat-sequence {
    tunnel: w15 -> [w310]
    tunnel: w14 -> [w309]
    tunnel: [w308] -> w13
    tunnel: [w312] -> w12
    tunnel: [w311] -> w11
    tunnel: w10 -> [w308]
    tunnel: [w307] -> w9
    tunnel: [w306] -> w8
    tunnel: w7 -> [w305]
    tunnel: [w304] -> w6
    tunnel: w13 -> [w351]
    tunnel: w12 -> [w352]
    tunnel: w11 -> [w353]
    tunnel: w9 -> [w350]
    tunnel: w8 -> [w349]
    tunnel: w6 -> [w348]
    frame #0 {
      n201 = while {
        tunnel: [w333] -> w312
        tunnel: w310 -> [w333]
        tunnel: w309 -> [w332]
        tunnel: [w332] -> w311
        tunnel: [w322] -> w307 mode=indexing
        tunnel: [w321] -> w306 mode=indexing
        tunnel: w305 -> [w320]
        tunnel: [w320] -> w304
        stop <- w313 stop-if-true
        w318 = u32 250 ("milliseconds to wait")
        w327 = 0.0 ("initial condition")
        n202 = local read "Drill-Z-stage Control"() -> (w323:refnum<k24>)
        n203 = local read "X-stage Control"() -> (w319:refnum<k24>)
        n204 = local read "Y-stage Control"() -> (w324:refnum<k24>)
        n205 = call "Y_absolute_position.vi"(".NET Refnum in"=w324) -> ("Numeric"=w326:dbl)  [unwired: 9 in, 1 out]
        n206 = call "Z_absolute_position.vi"(".NET Refnum in"=w323) -> ("Numeric"=w325:dbl)  [unwired: 9 in, 1 out]
        n207 = call "X-absolute_position.vi"(".NET Refnum in"=w319) -> ("Numeric"=w316:dbl)  [unwired: 9 in, 1 out]
        n208 = call <vilib>:"Derivative x(t) PtByPt.vi"("dt"=w318, "initial condition"=w327, "x"=w325) -> ("dx/dt"=w329:dbl)  [unwired: 1 in, 1 out]
        n209 = call <vilib>:"Derivative x(t) PtByPt.vi"("dt"=w318, "initial condition"=w327, "x"=w325) -> ("dx/dt"=w328:dbl)  [unwired: 1 in, 1 out]
        n210 = call <vilib>:"Derivative x(t) PtByPt.vi"("dt"=w318, "initial condition"=0.0, "x"=w316) -> ("dx/dt"=w315:dbl)  [unwired: 1 in, 1 out]
        n211 = Build Array(w325, w326, w316) -> (w321:dbl[])
        n212 = Build Array(w328, w329, w315) -> (w322:dbl[])
        n213 = Wait (ms)(milliseconds to wait=w318) -> ()  [unwired: 1 out]
        n214 = Array To Cluster(array=w321) -> (cluster=→"position":T1)
        n215 = Array To Cluster(array=w322) -> (cluster=→"Velocity":T1)
        n216 = case shown="True" "?" {
          tunnel: [FALSE w335] -> w313
          frame False {
          }
          frame True {
            n217 = flat-sequence {
              tunnel: [TRUE] -> w335
              frame #0 {
                n218 = local write "OCT ON"(TRUE ("OCT ON")) -> ()
                n219 = Wait (ms)(milliseconds to wait=u32 100) -> ()  [unwired: 1 out]
              }
              frame #1 {
                n220 = script code="close all\nclear camObject;"() -> ()  [unwired: 1 in, 1 out]
                n221 = call <vilib>:"System Exec.vi"("run minimized? (F)"=TRUE, "wait until completion? (T)"=TRUE, "command line"="cmd /c taskkill /IM OctEngine.exe") -> ()  [unwired: 5 in, 4 out]
              }
            }
          }
        }
      }
    }
    frame #1 {
      n222 = invoke class="KCubeDCServoControl" method="CloseDevice"(reference=w352) -> ()  [unwired: 2 in, 3 out]
      n223 = invoke class="BenchtopDCServoControl" method="CloseDevice"(reference=w353) -> ()  [unwired: 2 in, 3 out]
      n224 = invoke class="LongTravelStageControl" method="CloseDevice"(reference=w348) -> ()  [unwired: 2 in, 3 out]
      n225 = invoke class="KCubeDCServoControl" method="CloseDevice"(reference=w351) -> ()  [unwired: 2 in, 3 out]
      n226 = call <vilib>:"Application Directory.vi"() -> ("Application Directory"=w344:path)
      n227 = call <vilib>:"Application Directory.vi"() -> ("Application Directory"=w347:path)
      n228 = Build Path(base path=w344, name or relative path=path "velocity log.txt") -> (appended path=w342:path)
      n229 = call-poly <vilib>:"Write Delimited Spreadsheet.vi"("file path (dialog if empty)"=w342, "2D data"=w350) -> ()  [unwired: 12 in, 2 out]
      n230 = Build Path(base path=w347, name or relative path=path "position log.txt") -> (appended path=w345:path)
      n231 = call-poly <vilib>:"Write Delimited Spreadsheet.vi"("file path (dialog if empty)"=w345, "2D data"=w349) -> ()  [unwired: 12 in, 2 out]
    }
    frame #2 {
      n232 = Stop(stop? (T)=TRUE) -> ()
    }
  }
  n233 = local write "OCT ON"(FALSE) -> ()
  n234 = while {
    stop <- FALSE stop-if-true
    n235 = Wait (ms)(milliseconds to wait=u32 20) -> ()  [unwired: 1 out]
  }
  n236 = while {
    stop <- FALSE stop-if-true
    n237 = local read "OCT ON"() -> (w357:bool)
    n238 = case shown="True" w357 {
      frame False {
      }
      frame True {
        n239 = Concatenate Strings("OctEngine.exe" ("string"), "\r\n") -> (w365:string)
        n240 = call <vilib>:"System Exec.vi"("run minimized? (F)"=FALSE, "wait until completion? (T)"=TRUE, "working directory"=path "C:/Program Files/Lumedica/OctEngine", "standard input"=w365, "command line"="cmd /k cd C:\\Program Files\\Lumedica\\OctEngine ") -> ()  [unwired: 3 in, 4 out]
      }
    }
  }
